vi "SetAcquisitionModeSD.vi"(2 "error in (no error)":errorcluster, 3 "mode":T1=enum."Single Scan") -> (0 "error out":errorcluster, 1 "DLL error code":u32)   [LabVIEW 2015]
doc: "This function will set the acquisition mode to be used on the next <B>StartAcquisition</B>.\n\n<B>Parameter:</B>\nmode - the acquisition mode.\n Valid values: 0,5,7,8 Reserved DO NOT USE\n 1 - Single Scan\n 2 - Accumulate\n 3 - Kinetics\n 4 - Fast Kinetics\n 6 - Frame Transfer\n 9 - Time Delayed Integration (requires special files)\n\n<B>Error codes:</B>\nDRV_SUCCESS - Acquisition mode set.\nDRV_NOT_INITIALIZED - System not initialized.\nDRV_ACQUIRING - Acquisition in progress.\nDRV_P1INVALID - Acquisition Mode invalid.\n\n<B>NOTES:</B>\n<B>In modes 5 and 7 the system uses a \"Run Till Abort\" acquisition mode for non-Frame Transfer and Frame Transfer respectively. In these modes the camera continually acquires data until the AbortAcquisition function is called. These modes have not been tested under all conditions and hence are not listed above. You are free to try them. If you encounter any problem please notify us.</B>"
uses:
  AcquisitionMode_mode typedef.ctl
  DLL/atmcd32d.dll
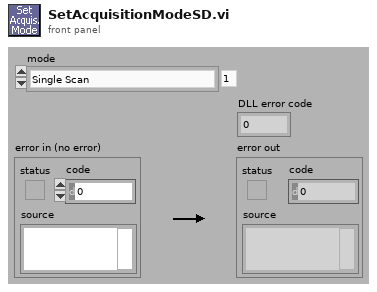
[diagram p1: front panel]
types:
  T1 = typedef "AcquisitionMode_mode typedef.ctl" = enum16{"Reserved (0)", "Single Scan", "Accumulate", "Kinetics", "Fast Kinetics", "Run Till Abort for non-Frame Transfer", "Frame Transfer", "Run Till Abort for Frame Transfer", "Reserved (8)", "Time Delayed Integration"}
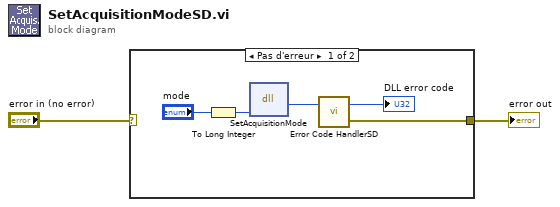
[diagram p0: block diagram]
diagram:
  n1 = case shown="Pas d'erreur" "error in (no error)" {
    selector: "error in (no error)" -> [_ w8]
    tunnel: [w6 w8] -> w1
    frame No Error {
      n2 = To Long Integer(number="mode") -> (32bit integer=w4:i32)
      n3 = dll-call lib="G:/SD/TRANCON/DLL/Atmcd32d.dll" fn="SetAcquisitionMode"("mode"=w4) -> (w7:u32)  [unwired: 4 in, 2 out]
      n4 = call "Error Code HandlerSD.vi"("DLL error code"=w7) -> ("error out"=w6:errorcluster, "dup DLL error code"=→"DLL error code":u32)  [unwired: 1 in]
    }
    frame Error {
    }
  }
  "error out" <- w1
